vi "GetRay.vi"(8 "error in (no error)":errorcluster, 10 "Point":T1, 11 "Control Window in":refnum<class "Control Window.lvclass">) -> (0 "error out":errorcluster, 1 "Far Point":T2, 2 "Near Point":T2, 3 "Control Window out":refnum<class "Control Window.lvclass">)   [LabVIEW 2015, in "Control Window.lvclass"]
uses:
  Control Window.lvclass
  <vilib>/Utility/miscctls.llb/LV3DPointTypeDef.ctl
  <vilib>/Utility/miscctls.llb/LVPoint32TypeDef.ctl
  Control Window.lvclass/Control Window.ctl
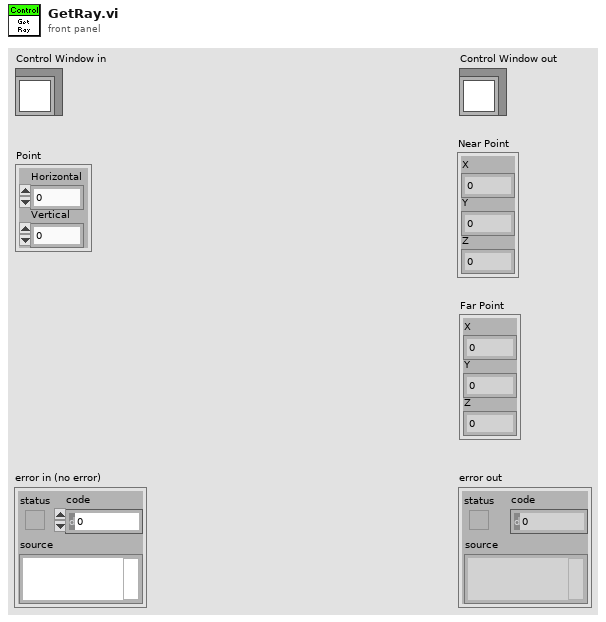
[diagram p1: front panel]
types:
  T1 = typedef "LVPoint32TypeDef.ctl" = cluster{"Horizontal":i32, "Vertical":i32}
  T2 = typedef "LV3DPointTypeDef.ctl" = cluster{"X":sgl, "Y":sgl, "Z":sgl}
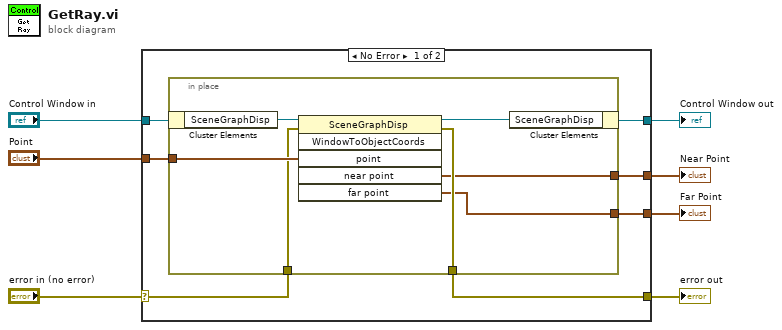
[diagram p0: block diagram]
diagram:
  n1 = case shown="No Error" "error in (no error)" {
    selector: "error in (no error)" -> [w12 w22]
    tunnel: [w11 w22] -> w6
    tunnel: "Control Window in" -> [w14 w23]
    tunnel: [w13 w23] -> w4
    tunnel: [w10 _] -> w3
    tunnel: [w9 _] -> w2
    tunnel: "Point" -> [w8 _]
    frame No Error {
      n2 = in-place {
        in-place-border: w12 -> [w15]
        in-place-border: [w20] -> w11
        in-place-border: [w19] -> w10
        in-place-border: [w18] -> w9
        in-place-border: w8 -> [w16]
        n3 = in-place-cluster #1(w14) -> ("SceneGraphDisp"=w17:refnum<vi>)
        n4 = invoke class="SceneGraphDisp" method="WindowToObjectCoords"(reference=w17, error in=w15, "point"=w16) -> (reference out=w21:refnum<vi>, error out=w20:errorcluster, "near point"=w19:T2, "far point"=w18:T2)  [unwired: 3 in, 2 out]
        n5 = in-place-cluster #1("SceneGraphDisp"=w21) -> (w13:refnum<class "Control Window.lvclass">)
      }
    }
    frame Error {
    }
  }
  "error out" <- w6
  "Control Window out" <- w4
  "Near Point" <- w3
  "Far Point" <- w2
